vi "PathPlanner_Cmd_FollowLTVUnicyclePathExecute.vi"(5 "PathPlanner_Cmd_FollowLTVUnicycleConfig":T17={"ControlPastEnd_Sec"=3.0, "ReplanningConfig"={"enableInitialReplanning"=TRUE, "enableDynamicReplanning"=FALSE, "dynamicReplanningTotalErrorThreshold"=1.0, "dynamicReplanningErrorSpikeThreshold"=0.25}, "Trigger Events"=TRUE, "LTV_Unicycle_Ctrl_Model"={"Max linear ctrl effort M/S"=2.0, "Max angular ctrl effort Rad/S"=0.7, "Max Heading Meas Tol Rad"=2.0, "Max X Pos Meas Tol M"=0.7, "Max Y Pos Meas Tol M"=0.7, "Max Linear Vel M/S"=2.0}, "X Tolerance M"=0.0762, "Y Tolerance M"=0.0762, "Rotation Tolerance DEG"=0.0872665, "Track Width Meters"=1.0, "Max Speed M/S"=4.0, "Period"=0.02} {"LTV_Unicycle_Ctrl_Model"."Max Linear Vel M/S" format="%#_13g"; "LTV_Unicycle_Ctrl_Model"."Max Y Pos Meas Tol M" format="%#_13g"; "LTV_Unicycle_Ctrl_Model"."Max X Pos Meas Tol M" format="%#_13g"; "LTV_Unicycle_Ctrl_Model"."Max Heading Meas Tol Rad" format="%#_13g"; "LTV_Unicycle_Ctrl_Model"."Max angular ctrl effort Rad/S" format="%#_13g"; "LTV_Unicycle_Ctrl_Model"."Max linear ctrl effort M/S" format="%#_13g"}, 6 "PassthroughTime_SEC":dbl=-1.0, 7 "PathPlannerPath":T8={"BezierPoints"=[], "PreviewStartingRotation"={"VALUE"=0.0, "COS"=1.0, "SIN"=0.0}, "Reversed"=FALSE, "RotationTargets"=[], "ConstraintZones"=[], "EventMarkers"=[], "GlobalConstraints"={"MaxVelocityMps;"=0.0, "MaxAccelerationMpsSq;"=0.0, "MaxAngularVelRadPsEc;"=0.0, "MaxAngularAccRadPSecSq"=0.0, "Exists"=FALSE}, "GoalEndState"={"Velocity"=0.0, "Rotation"={"VALUE"=0.0, "COS"=1.0, "SIN"=0.0}}, "AllPoints"=[]} {"AllPoints"."HolonomicRotation"."SIN" format="%13.4f"; "AllPoints"."HolonomicRotation"."COS" format="%13.4f"; "AllPoints"."HolonomicRotation"."VALUE" format="%13.4f"; "AllPoints"."Position"."Y" format="%14.3f"; "AllPoints"."Position"."X" format="%14.3f"; "GoalEndState"."Rotation"."SIN" format="%13.4f"; "GoalEndState"."Rotation"."COS" format="%13.4f"; "GoalEndState"."Rotation"."VALUE" format="%13.4f"; "EventMarkers"."lastRobotPos"."Y" format="%14.3f"; "EventMarkers"."lastRobotPos"."X" format="%14.3f"; "EventMarkers"."markerPos"."Y" format="%14.3f"; "EventMarkers"."markerPos"."X" format="%14.3f"; "RotationTargets"."target"."SIN" format="%13.4f"; "RotationTargets"."target"."COS" format="%13.4f"; "RotationTargets"."target"."VALUE" format="%13.4f"; "PreviewStartingRotation"."SIN" format="%13.4f"; "PreviewStartingRotation"."COS" format="%13.4f"; "PreviewStartingRotation"."VALUE" format="%13.4f"; "BezierPoints"."Y" format="%14.3f"; "BezierPoints"."X" format="%14.3f"}, 8 "Enabled":bool=TRUE, 9 "Reset":bool, 10 "CurrentChassisSpeeds":T7 {"vOmega" format="%10.3f"; "vY" format="%10.3f"; "vX" format="%10.3f"}, 11 "Current Pose SI":T2={"TRANSLATION"={"X"=0.0, "Y"=0.0}, "ROTATION"={"VALUE"=0.0, "COS"=1.0, "SIN"=0.0}} {"ROTATION"."SIN" format="%13.4f"; "ROTATION"."COS" format="%13.4f"; "ROTATION"."VALUE" format="%13.4f"; "TRANSLATION"."Y" format="%14.3f"; "TRANSLATION"."X" format="%14.3f"}) -> (0 "Position Error M":dbl, 1 "Complete":bool, 2 "At Reference":bool, 3 "Left Right Speed Dmds":T6, 4 "out LTV_UNICYCLE_CONTROLLER":T1={"States"=3, "Inputs"=2, "PoseError"={"TRANSLATION"={"X"=0.0, "Y"=0.0}, "ROTATION"={"VALUE"=0.0, "COS"=1.0, "SIN"=0.0}}, "PoseTolerance"={"TRANSLATION"={"X"=0.0, "Y"=0.0}, "ROTATION"={"VALUE"=0.0, "COS"=1.0, "SIN"=0.0}}, "Dt"=0.02, "Enabled"=TRUE, "LQR_K_Table"={"Table Xs"=[], "Table Ys"=[], "MinX"=0.0, "MaxX"=0.0, "ItemCount"=0, "Rows"=0, "Columns"=0}} {"PoseTolerance"."ROTATION"."SIN" format="%13.4f"; "PoseTolerance"."ROTATION"."COS" format="%13.4f"; "PoseTolerance"."ROTATION"."VALUE" format="%13.4f"; "PoseTolerance"."TRANSLATION"."Y" format="%14.3f"; "PoseTolerance"."TRANSLATION"."X" format="%14.3f"; "PoseError"."ROTATION"."SIN" format="%13.4f"; "PoseError"."ROTATION"."COS" format="%13.4f"; "PoseError"."ROTATION"."VALUE" format="%13.4f"; "PoseError"."TRANSLATION"."Y" format="%14.3f"; "PoseError"."TRANSLATION"."X" format="%14.3f"})   [LabVIEW 2019, in "PathPlanner24.lvlib"]
doc: "Calculates the next output of the path following controller for holonomic drive robots. This wraps a Holonomic Drive Control function with the particulars needed to follow a PathPlanner trajectory.\n\nInputs:\n - PathPlanner_Holonomic_Ctrl_Pack_Tuning - cluster - The tuning paraameters for the holonomic drive controller. These are static. They should not be changed after the first call to this function.\n - CurrentPoseSi - pose2d - The current pose calculated by odometry or pose estimation. The pose can be absolute or relative depending on what type of trajectory is being followed.\n - PathPlannerState - cluster - The path palnner trajectory state containing the desired position and velocities of the robot.\n - Reset - boolean - When TRUE the holonomic drive controller is reset. This should be set to TRUE for the first execution of a trajectory.\n - Enabled - boolean - When TRUE, closed loop control is enabled. (Optional. Default: TRUE)\n - Period - double - The loop period in seconds for this controller. (Optional. Default: 0.020)\n\nOutputs:\n - CalcChassisSpeed - cluster - The desired chassis speed in SI units.\n - AtReference - boolean - TRUE if the robots position is within the defined tolerance.\n - PositionError - pose2d - Position error in SI units. How far the robot is away from the desired trajectory position.\n - out_Holonomic_Drive_Ctrl - THe current holonomic drive controller data cluster. This is mainly for diagnostic purposes."
uses:
  PathPlanner24.lvlib
  <vilib>/Rock Robotics/WPI/ThirdParty/JAS_Junk/TrajLib/TypeDef/POSE2D.ctl
  <vilib>/Rock Robotics/WPI/ThirdParty/JAS_Junk/TrajLib/TypeDef/TRANSLATION2D.ctl
  <vilib>/Rock Robotics/WPI/ThirdParty/JAS_Junk/TrajLib/TypeDef/ROTATION2D.ctl
  TypeDef/PathPlannerCmdFollowLTVUnicycleConfig.ctl
  TypeDef/PathPlannerReplanningConfig.ctl
  <vilib>/Rock Robotics/WPI/ThirdParty/JAS_Junk/TrajLib/TypeDef/LTV_UNICYCLE_CONTROLLER_MODEL_PARAMS.CTL
  TypeDef/PathPlannerPath.ctl
  TypeDef/PathPlannerRotationTarget.ctl
  TypeDef/PathPlannerConstraintsZone.ctl
  TypeDef/PathPlannerPathConstraints.ctl
  TypeDef/PathPlannerEventMarker.ctl
  TypeDef/PathPlannerCommandUtil.ctl
  ENum/PathPlanner_CommandUtilType_ENUM.ctl
  TypeDef/PathPlannerGoalEndState.ctl
  TypeDef/PathPlannerPathPoint.ctl
  <vilib>/Rock Robotics/WPI/ThirdParty/JAS_Junk/TrajLib/TypeDef/CHASSIS_SPEEDS.ctl
  <vilib>/Rock Robotics/WPI/ThirdParty/JAS_Junk/TrajLib/TypeDef/LTV_UNICYCLE_CONTROLLER.ctl
  <vilib>/Rock Robotics/WPI/ThirdParty/JAS_Junk/TrajLib/TypeDef/FUNCTION_GENERATOR_MATRIX.ctl
  PathPlanner_EventMarker_Reset.vi
  <vilib>/Rock Robotics/WPI/ThirdParty/JAS_Junk/TrajLib/Conv_Deg_Radians.vi
  <vilib>/Rock Robotics/WPI/ThirdParty/JAS_Junk/TrajLib/Pose2d_getTranslation.vi
  <vilib>/Rock Robotics/WPI/ThirdParty/JAS_Junk/TrajLib/Trajectory_Library.lvlib
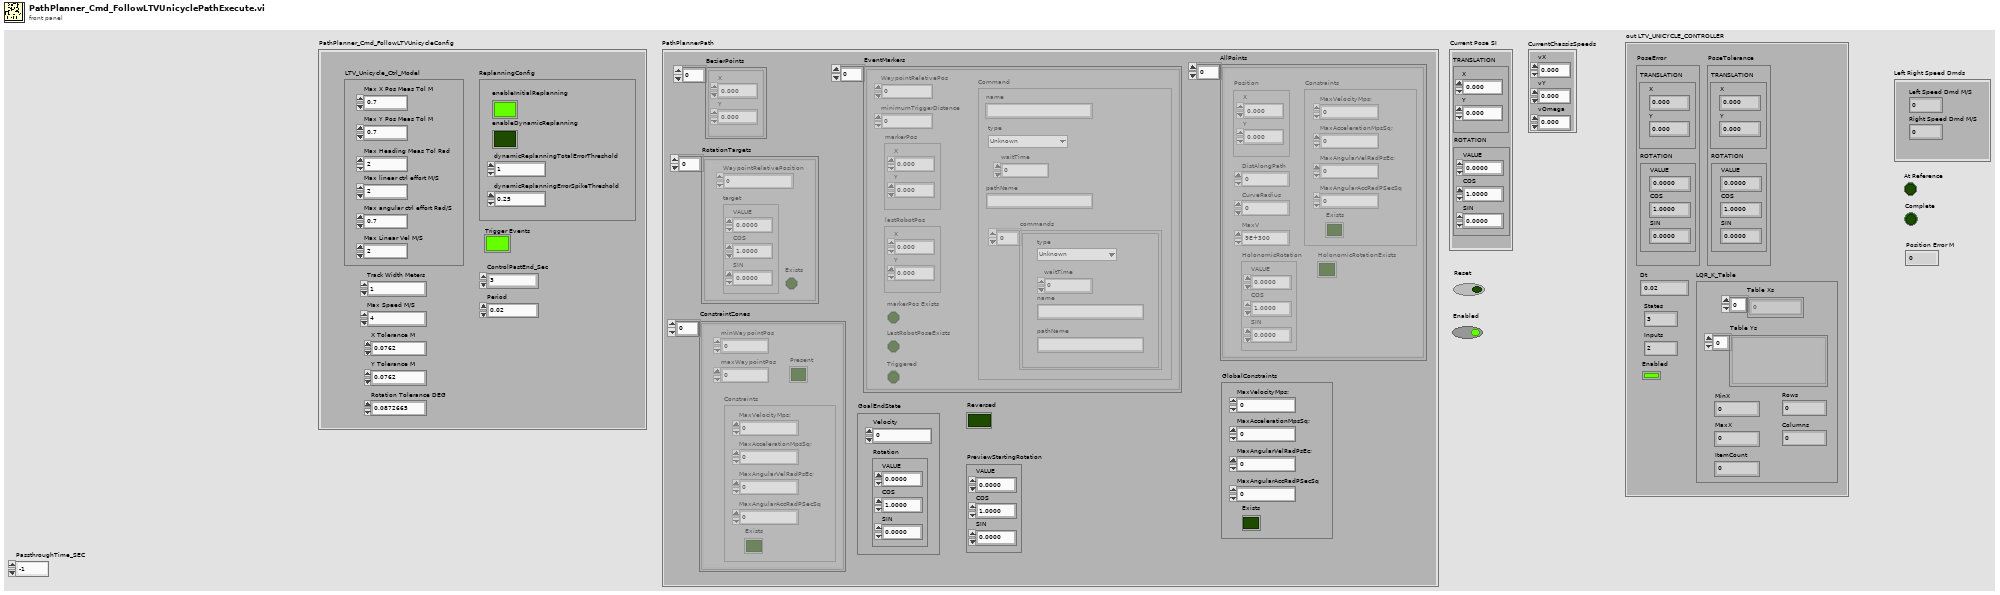
[diagram p1: front panel]
types:
  T1 = typedef "Trajectory_Library.lvlib/LTV_UNICYCLE_CONTROLLER.ctl" = cluster{"States":i32, "Inputs":i32, "PoseError":T2, "PoseTolerance":T2, "Dt":dbl, "Enabled":bool, "LQR_K_Table":T5}
  T2 = typedef "Trajectory_Library.lvlib/POSE2D.ctl" = cluster{"TRANSLATION":T3, "ROTATION":T4}
  T3 = typedef "Trajectory_Library.lvlib/TRANSLATION2D.ctl" = cluster{"X":dbl, "Y":dbl}
  T4 = typedef "Trajectory_Library.lvlib/ROTATION2D.ctl" = cluster{"VALUE":dbl, "COS":dbl, "SIN":dbl}
  T5 = typedef "Trajectory_Library.lvlib/FUNCTION_GENERATOR_MATRIX.ctl" = cluster{"Table Xs":dbl[], "Table Ys":variant[], "MinX":dbl, "MaxX":dbl, "ItemCount":i32, "Rows":i32, "Columns":i32}
  T6 = cluster{"Left Speed Dmd M/S":dbl, "Right Speed Dmd M/S":dbl}
  T7 = typedef "Trajectory_Library.lvlib/CHASSIS_SPEEDS.ctl" = cluster{"vX":dbl, "vY":dbl, "vOmega":dbl}
  T8 = typedef "PathPlanner24.lvlib/PathPlannerPath.ctl" = cluster{"BezierPoints":T3[], "PreviewStartingRotation":T4, "Reversed":bool, "RotationTargets":T9[], "ConstraintZones":T10[], "EventMarkers":T12[], "GlobalConstraints":T11, "GoalEndState":T15, "AllPoints":T16[]}
  T9 = typedef "PathPlanner24.lvlib/PathPlannerRotationTarget.ctl" = cluster{"target":T4, "WaypointRelativePosition":dbl, "Exists":bool}
  T10 = typedef "PathPlanner24.lvlib/PathPlannerConstraintsZone.ctl" = cluster{"minWaypointPos":dbl, "maxWaypointPos":dbl, "Constraints":T11, "Present":bool}
  T11 = typedef "PathPlanner24.lvlib/PathPlannerPathConstraints.ctl" = cluster{"MaxVelocityMps;":dbl, "MaxAccelerationMpsSq;":dbl, "MaxAngularVelRadPsEc;":dbl, "MaxAngularAccRadPSecSq":dbl, "Exists":bool}
  T12 = typedef "PathPlanner24.lvlib/PathPlannerEventMarker.ctl" = cluster{"WaypointRelativePos":dbl, "minimumTriggerDistance":dbl, "markerPos":T3, "lastRobotPos":T3, "Command":T13, "markerPos Exists":bool, "LastRobotPoseExists":bool, "Triggered":bool}
  T13 = typedef "PathPlanner24.lvlib/PathPlannerCommandUtil.ctl" = cluster{"waitTime":dbl, "name":string, "pathName":string, "commands":cluster{"type":T14, "waitTime":dbl, "name":string, "pathName":string}[], "type":T14}
  T14 = typedef "PathPlanner24.lvlib/PathPlanner_CommandUtilType_ENUM.ctl" = enum16{"Unknown", "Wait", "Named", "Path", "Sequential", "Parallel", "Race", "Deadline"}
  T15 = typedef "PathPlanner24.lvlib/PathPlannerGoalEndState.ctl" = cluster{"Velocity":dbl, "Rotation":T4}
  T16 = typedef "PathPlanner24.lvlib/PathPlannerPathPoint.ctl" = cluster{"Position":T3, "HolonomicRotation":T4, "DistAlongPath":dbl, "CurveRadius":dbl, "MaxV":dbl, "Constraints":T11, "HolonomicRotationExists":bool}
  T17 = typedef "PathPlanner24.lvlib/PathPlannerCmdFollowLTVUnicycleConfig.ctl" = cluster{"ControlPastEnd_Sec":dbl, "ReplanningConfig":T18, "Trigger Events":bool, "LTV_Unicycle_Ctrl_Model":T19, "X Tolerance M":dbl, "Y Tolerance M":dbl, "Rotation Tolerance DEG":dbl, "Track Width Meters":dbl, "Max Speed M/S":dbl, "Period":dbl}
  T18 = typedef "PathPlanner24.lvlib/PathPlannerReplanningConfig.ctl" = cluster{"enableInitialReplanning":bool, "enableDynamicReplanning":bool, "dynamicReplanningTotalErrorThreshold":dbl, "dynamicReplanningErrorSpikeThreshold":dbl}
  T19 = typedef "Trajectory_Library.lvlib/LTV_UNICYCLE_CONTROLLER_MODEL_PARAMS.CTL" = cluster{"Max linear ctrl effort M/S":dbl, "Max angular ctrl effort Rad/S":dbl, "Max Heading Meas Tol Rad":dbl, "Max X Pos Meas Tol M":dbl, "Max Y Pos Meas Tol M":dbl, "Max Linear Vel M/S":dbl}
  T20 = typedef "PathPlanner24.lvlib/PathPlannerCtrlLTVUnicycleConfig.ctl" = cluster{"Max Wheel Speed M/S":dbl, "Track Width M":dbl, "LTV_Unicycle_Ctrl_Model":T19, "LTV_Unicycle_Ctrl_Tolerance":T21}
  T21 = typedef "Trajectory_Library.lvlib/LTV_UNICYCLE_CONTROLLER_TOLERANCE.CTL" = cluster{"Max Heading Tolerance Rad":dbl, "Max X Tolerance M":dbl, "Max Y Tolerance M":dbl}
  T22 = cluster{"Traj Time Plus Extra\nElapsed":bool, "Traj Time Elapsed":bool}
  T23 = typedef "PathPlanner24.lvlib/PathPlannerTrajectoryState.ctl" = cluster{"TimeSeconds":dbl, "VelocityMPS":dbl, "AccerationMpsSq":dbl, "HeadingAngularVelRadPerSec":dbl, "PositionMeters":T3, "Heading":T4, "TargetHolonomicRotation":T4, "CurvatureRadPerMeter":dbl, "PathPlannerConstraints":T11, "DeltaPos":dbl}
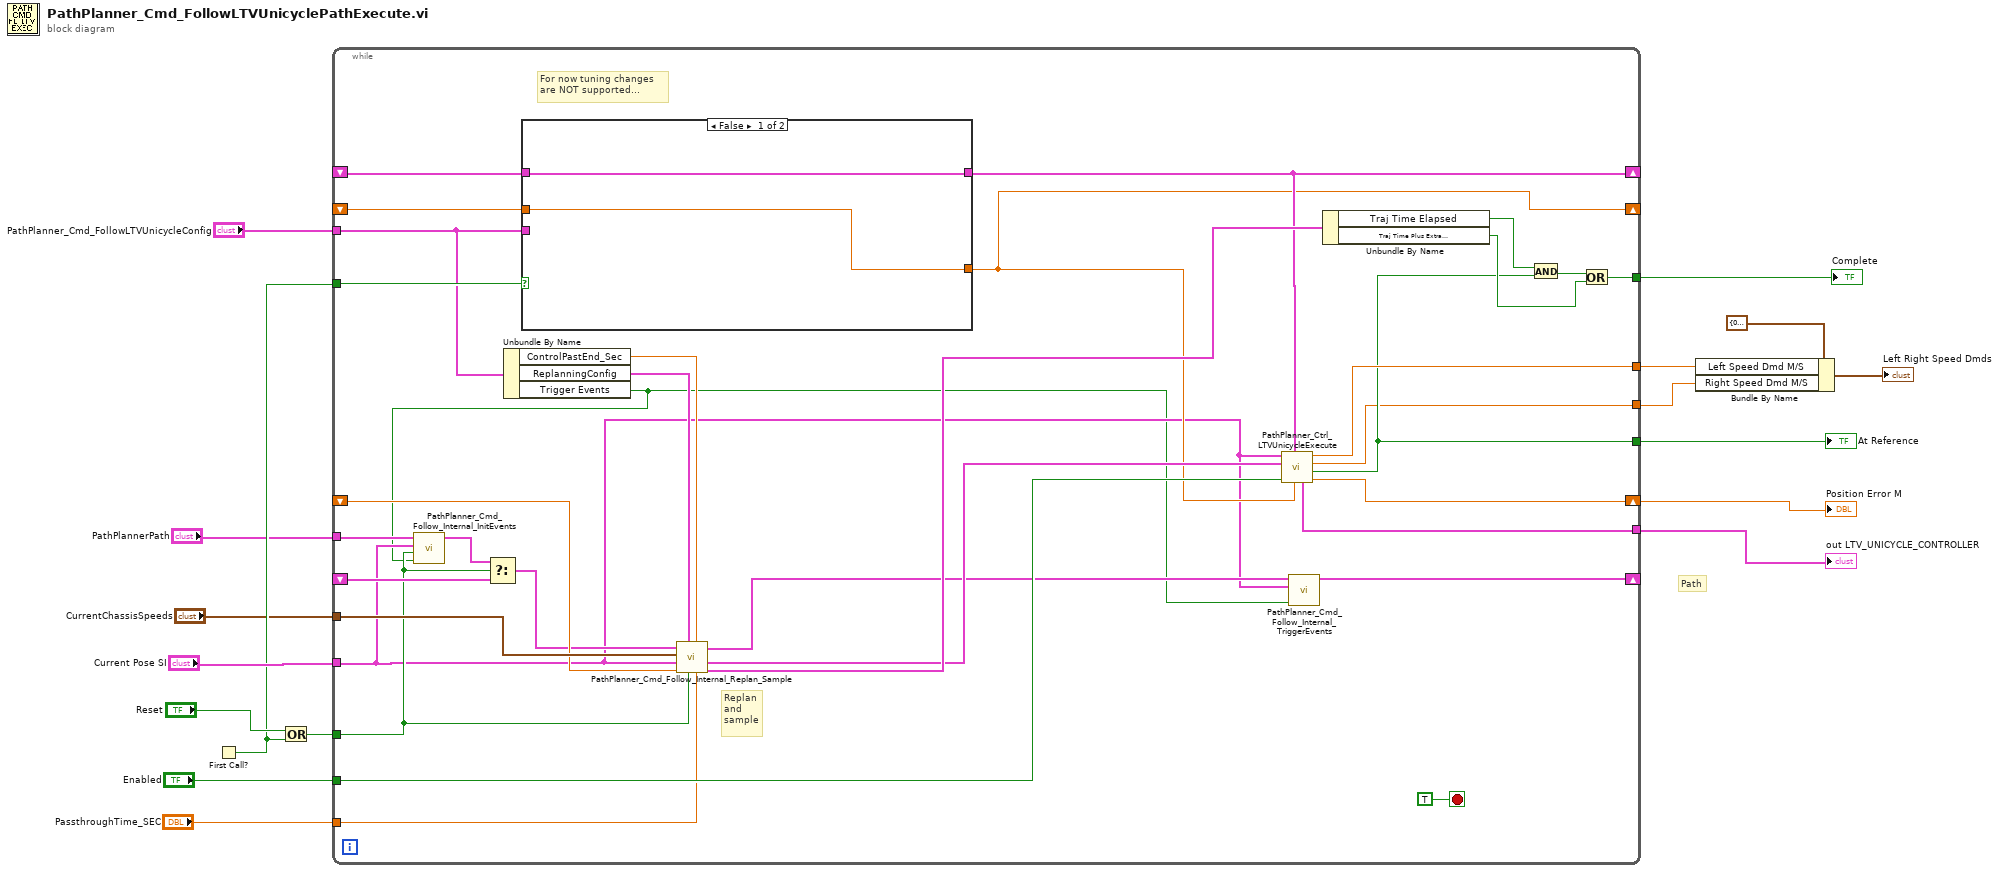
[diagram p0: block diagram]
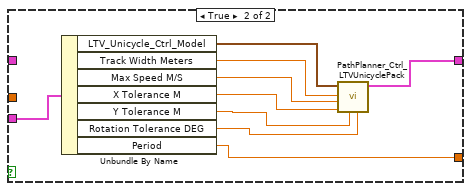
[diagram p2: hidden frame]
diagram:
  # "Path"
  n1 = First Call?() -> (First Call?: T/F=w11:bool)
  n2 = Or(x="Reset", y=w11) -> (x .or. y?=w13:bool)
  n3 = while {
    tunnel: "PathPlanner_Cmd_FollowLTVUnicycleConfig" -> [w39]
    tunnel: "Current Pose SI" -> [w19]
    tunnel: w11 -> [w50]
    shift-right: [w27] -> _
    shift-left: _ -> [w48]
    tunnel: "Enabled" -> [w47]
    tunnel: [w31] -> w12
    tunnel: "CurrentChassisSpeeds" -> [w44]
    shift-right: [w20] -> _
    shift-left: _ -> [w40]
    tunnel: "PassthroughTime_SEC" -> [w43]
    tunnel: [w45] -> w1
    shift-right: [w46] -> w9
    shift-left: _ -> [w42]
    tunnel: w13 -> [w22]
    tunnel: "PathPlannerPath" -> [w23]
    tunnel: [w36] -> w6
    tunnel: [w32] -> w3
    tunnel: [w30] -> w2
    shift-right: [w25] -> _
    shift-left: _ -> [w26]
    stop <- TRUE stop-if-true
    # "Replan\nand \nsample"
    # "For now tuning changes\nare NOT supported..."
    n4 = Unbundle By Name(w39) -> ("ControlPastEnd_Sec"=w28:dbl, "ReplanningConfig"=w38:T18, "Trigger Events"=w18:bool)
    n5 = call "PathPlanner_Cmd_Follow_Internal_InitEvents.vi"("TrigerEvents"=w18, "Reset In"=w22, "Current Pose SI"=w19, "RePlannedPath in"=w23) -> ("RePlannedPath out"=w24:T8)  [unwired: 7 in]
    n6 = Select(t=w24, s=w22, f=w40) -> (s? t:f=w41:T8)
    n7 = case shown="False" w50 {
      tunnel: [w52 w61] -> w27
      tunnel: w39 -> [_ w60]
      tunnel: w48 -> [w52 _]
      tunnel: [w51 w53] -> w25
      tunnel: w26 -> [w51 _]
      frame False {
      }
      frame True {
        n8 = Unbundle By Name(w60) -> ("LTV_Unicycle_Ctrl_Model"=w59:T19, "Track Width Meters"=w58:dbl, "Max Speed M/S"=w57:dbl, "X Tolerance M"=w56:dbl, "Y Tolerance M"=w55:dbl, "Rotation Tolerance DEG"=w54:dbl, "Period"=w53:dbl)
        n9 = call "PathPlanner_Ctrl_LTVUnicyclePack.vi"("Rotation Tolerance DEG"=w54, "Y Tolerance M"=w55, "X Tolerance M"=w56, "Max Speed M/S"=w57, "Track Width Meters"=w58, "LTV_Unicycle_Ctrl_Model"=w59) -> ("PathPlanner_Ctrl_LTVUnicycleConfig"=w61:T20)  [unwired: 5 in]
      }
    }
    n10 = call "PathPlanner_Cmd_Follow_Internal_Replan_Sample.vi"("PassthroughTime_SEC"=w43, "Extra Time Sec"=w28, "Reset In"=w22, "ReplanningConfig"=w38, "Position Error M"=w42, "Current Pose SI"=w19, "CurrentChassisSpeeds"=w44, "RePlannedPath in"=w41) -> ("Traj End Status"=w35:T22, "Trajectory State"=w29:T23, "RePlannedPath out"=w21:T8)  [unwired: 1 out]
    n11 = call "PathPlanner_Ctrl_LTVUnicycleExecute.vi"("Period"=w25, "PathPlanner_Ctrl_LTVUnicycle_Config"=w27, "Enabled"=w47, "PathPlannerState"=w29, "Current Pose SI"=w19) -> ("Position Error M"=w46:dbl, "At Reference"=w31:bool, "Normalized Right Wheel Dmd M/S"=w30:dbl, "Normalized Left Wheel Dmd M/S"=w32:dbl, "out LTV_UNICYCLE_CONTROLLER"=w45:T1)  [unwired: 2 in]
    n12 = call "PathPlanner_Cmd_Follow_Internal_TriggerEvents.vi"("TrigerEvents"=w18, "Current Pose SI"=w19, "RePlannedPath in"=w21) -> ("RePlannedPath out"=w20:T8)  [unwired: 8 in]
    n13 = Unbundle By Name(w35) -> ("Traj Time Elapsed"=w34:bool, "Traj Time Plus Extra\nElapsed"=w33:bool)
    n14 = And(x=w34, y=w31) -> (x .and. y?=w37:bool)
    n15 = Or(x=w37, y=w33) -> (x .or. y?=w36:bool)
  }
  "At Reference" <- w12
  "Position Error M" <- w9
  "Complete" <- w6
  "out LTV_UNICYCLE_CONTROLLER" <- w1
  n16 = Bundle By Name(cluster=T6 {"Left Speed Dmd M/S"=0.0, "Right Speed Dmd M/S"=0.0} ("Left Right Speed Dmds"), "Left Speed Dmd M/S"=w3, "Right Speed Dmd M/S"=w2) -> (→"Left Right Speed Dmds":T6)
